vi "小波分析多尺度峰值检测.vi"() -> ()   [LabVIEW 2015]
uses:
  <vilib>/addons/Wavelet Analysis/application.llb/WA Multiscale Peak Detection (Array).vi
  <vilib>/addons/_Advanced Signal Processing/NI_AdvSigProcWA.lvlib
panel:
  in  "sampling rate":dbl=1.0 format="%#_13g"
  in  "detrend settings":T1={"detrend? (F)"=FALSE, "threshold frequency"=-1.0}
  in  "threshold":dbl=1.5 format="%#_13g"
  in  "width":i32=3
  out "peak plot":cluster{"Ramp Pattern":dbl[], "X":dbl[]}[](graph)
  out "amplitude":dbl[](array[numeric])
  out "location":dbl[](array[numeric])
  out "number of peaks":i32
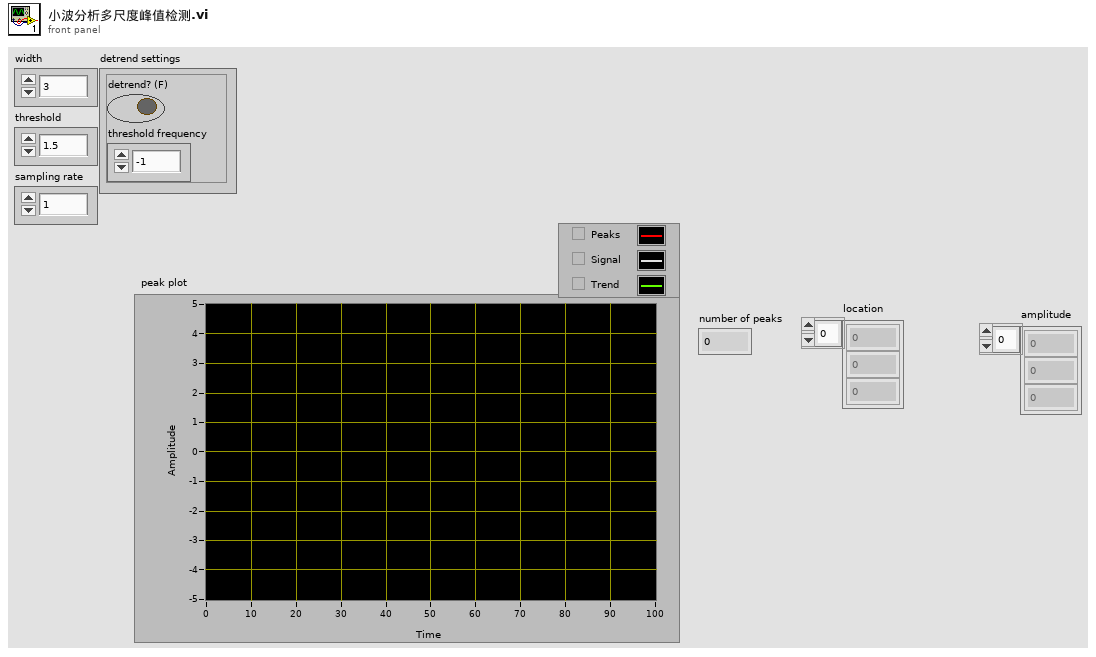
[diagram p1: front panel]
types:
  T1 = cluster{"detrend? (F)":bool, "threshold frequency":dbl}
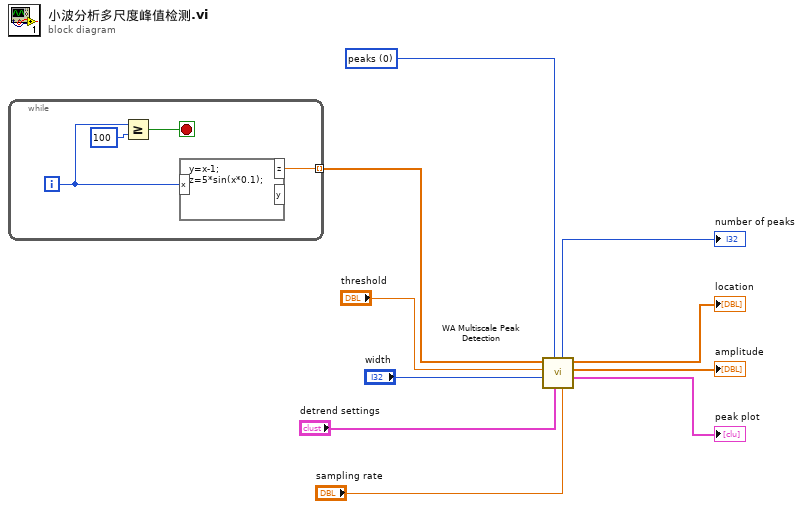
[diagram p0: block diagram]
diagram:
  w2 = u16 0 items=["peaks", "valleys"] ("peaks/valleys")
  n1 = while {
    tunnel: [w11] -> w1 mode=indexing
    i -> [w14]
    stop <- w12 stop-if-true
    n2 = Greater Or Equal?(x=w14, y=100) -> (x >= y?=w12:bool)
    n3 = formula code="y=x-1;\nz=5*sin(x*0.1);"("x"=w14) -> ("z"=w11:dbl)  [unwired: 1 out]
  }
  n4 = call-poly <vilib>:"WA Multiscale Peak Detection.vi"("sampling rate"="sampling rate", "detrend settings"="detrend settings", "peaks/valleys"=w2, "width"="width", "threshold"="threshold", "signal"=w1) -> ("peak plot"=→"peak plot":cluster{"Ramp Pattern":dbl[], "X":dbl[]}[], "amplitude"=→"amplitude":dbl[], "location"=→"location":dbl[], "number of peaks"=→"number of peaks":i32)  [unwired: 1 in, 1 out]
